vi "Autosetup.vi"(8 "error in (no error)":errorcluster, 11 "EDUX1002G in":refnum<class "EDUX1002G.lvclass">) -> (0 "error out":errorcluster, 3 "EDUX1002G out":refnum<class "EDUX1002G.lvclass">)   [LabVIEW 2020, in "Osciloscope Tektronix.lvlib" / "EDUX1002G.lvclass"]
uses:
  EDUX1002G.lvclass
  C:/Users/Pablo/Osciloscope-Tek/TDS2000/Libraries/Osciloscope Tektronix/Clases/Osciloscope/Osciloscope.lvclass
  Osciloscope/Osciloscope.lvclass/Osciloscope.ctl
  Osciloscope/Read COM.vi
  <instrlib>/Agilent 2000 3000 X-Series/Agilent 2000 3000 X-Series.lvlib
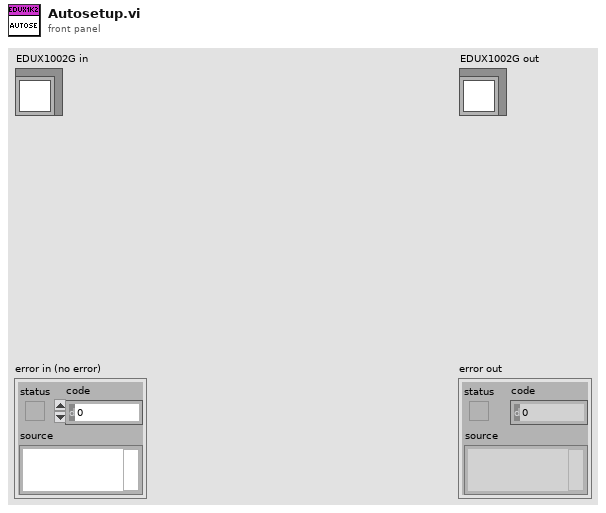
[diagram p1: front panel]
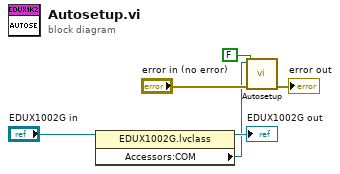
[diagram p0: block diagram]
diagram:
  n1 = property class="EDUX1002G.lvclass"(reference="EDUX1002G in") -> (reference out=→"EDUX1002G out":refnum<class "EDUX1002G.lvclass">, "Accessors:COM"=w2:refnum<visa-resource-name>)  [unwired: 1 in, 1 out]
  n2 = call <instrlib>:"Autosetup.vi"("error in (no error)"="error in (no error)", "Enable Fast Debug Auto Scaling (F: Disable)"=FALSE, "VISA resource name"=w2) -> ("error out"=→"error out":errorcluster)  [unwired: 7 in, 1 out]
